vi "RT_Delta.vi"(4 "2812 -A Params In":T12={"Auto Range?"=FALSE, "Man / Selected\nRange"=enum."10mV", "Enable Digital\nFilter?"=FALSE, "Filter Type"=enum."Moving", "Filter Count"=10, "Filter\nWindow (%)"=0.01, "Enable Analog\nFilter?"=FALSE, "NPLCs"=5} {"Filter\nWindow (%)" min=0.0 max=10.0 step=0.01 format="%.2f"; "Filter Count" min=1 max=100; "NPLCs" min=1 max=10}, 6 "Delta Mode Params In":T1={"High Level (A)"=0.001, "Low Level (A)"=-0.001, "Delay (s)"=0.002, "Num Cycles Mode"=enum."Finite Count", "Finite Count"=10, "Abort On\nCompliance?"=FALSE, "Cold Swithing\nMode Enabled?"=FALSE} {"Finite Count" min=2 max=65536; "Low Level (A)" min=-0.105 max=0.0 format="%.3p"; "High Level (A)" min=0.0 max=0.105 format="%.3p"; "Delay (s)" min=0.001 max=9999.999 format="%.3f"}, 8 "error in (no error)":errorcluster, 11 "Resource In":refnum<visa-resource-name>) -> (0 "error out":errorcluster, 1 "Current (A)":sgl, 2 "Voltage (V)":dbl format="%0.2f", 3 "Resource Out (dupl)":refnum<visa-resource-name>)   [LabVIEW 2024]
uses:
  <instrlib>/Keithley 622x LV 2009/Configure/2182 -A/Low Level/Typedefs/KE2182 -- Voltage Ranges.ctl
  <instrlib>/Keithley 622x LV 2009/Configure/2182 -A/Low Level/Typedefs/KE2182 -- Filter Type.ctl
  <instrlib>/Keithley 622x LV 2009/Configure/2182 -A/Low Level/Typedefs/KE2182 -- Filter Count.ctl
  <instrlib>/Keithley 622x LV 2009/Configure/2182 -A/Low Level/Typedefs/KE2182 -- Filter Window.ctl
  <instrlib>/Keithley 622x LV 2009/Configure/2182 -A/Low Level/Typedefs/KE2182 -- NPLCs.ctl
  <instrlib>/Keithley 622x LV 2009/Configure/Delta PDelta DCon Modes/Typedefs/KE622x -- Delta Mode Params.ctl
  <instrlib>/Keithley 622x LV 2009/Configure/Delta PDelta DCon Modes/Low Level/Typedefs/KE622x -- Delta PDelta Mode High Level.ctl
  <instrlib>/Keithley 622x LV 2009/Configure/Delta PDelta DCon Modes/Low Level/Typedefs/KE622x -- Delta PDelta Mode Low Level.ctl
  <instrlib>/Keithley 622x LV 2009/Configure/Delta PDelta DCon Modes/Low Level/Typedefs/KE622x -- Delta DCon Mode Delay.ctl
  <instrlib>/Keithley 622x LV 2009/Configure/Delta PDelta DCon Modes/Low Level/Typedefs/KE622x -- Delta PDelta Mode Num Cycles Mode.ctl
  <instrlib>/Keithley 622x LV 2009/Configure/Delta PDelta DCon Modes/Low Level/Typedefs/KE622x -- Delta PDelta Mode Num Cycles.ctl
  <instrlib>/Keithley 622x LV 2009/Configure/Format/Typedefs/KE622x -- Optional Meas Elements.ctl
  <instrlib>/Keithley 622x LV 2009/Configure/Units/Typedefs/KE622x -- Voltage Meas Units.ctl
  <vilib>/Analysis/baseanly.llb/Mean (DBL).vi
  <instrlib>/Keithley 622x LV 2009/Keithley 622x.lvlib
  <vilib>/Analysis/NI_AALBase.lvlib
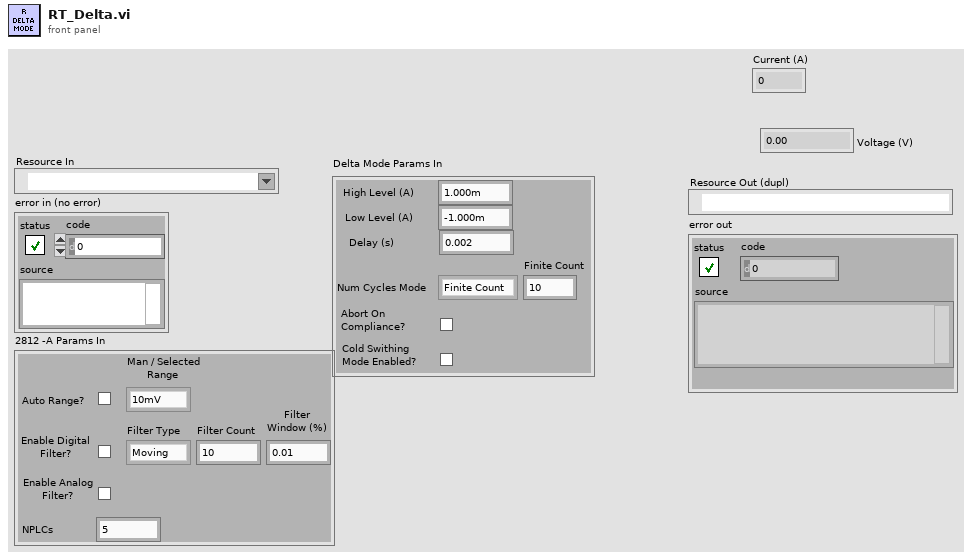
[diagram p1: front panel]
types:
  T1 = typedef "Keithley 622x.lvlib/KE622x -- Delta Mode Params.ctl" = cluster{"High Level (A)":T2, "Low Level (A)":T3, "Delay (s)":T4, "Num Cycles Mode":T5, "Finite Count":T6, "Abort On\nCompliance?":bool, "Cold Swithing\nMode Enabled?":bool}
  T2 = typedef "Keithley 622x.lvlib/KE622x -- Delta PDelta Mode High Level.ctl" = dbl
  T3 = typedef "Keithley 622x.lvlib/KE622x -- Delta PDelta Mode Low Level.ctl" = dbl
  T4 = typedef "Keithley 622x.lvlib/KE622x -- Delta DCon Mode Delay.ctl" = dbl
  T5 = typedef "Keithley 622x.lvlib/KE622x -- Delta PDelta Mode Num Cycles Mode.ctl" = enum16{"Finite Count", "Infinite"}
  T6 = typedef "Keithley 622x.lvlib/KE622x -- Delta PDelta Mode Num Cycles.ctl" = u32
  T7 = typedef "Keithley 622x.lvlib/KE2182 -- Voltage Ranges.ctl" = enum16{"10mV", "100mV", "1V", "10V", "100V"}
  T8 = typedef "Keithley 622x.lvlib/KE2182 -- Filter Type.ctl" = enum16{"Moving", "Repeat"}
  T9 = typedef "Keithley 622x.lvlib/KE2182 -- Filter Count.ctl" = u32
  T10 = typedef "Keithley 622x.lvlib/KE2182 -- Filter Window.ctl" = dbl
  T11 = typedef "Keithley 622x.lvlib/KE2182 -- NPLCs.ctl" = u32
  T12 = cluster{"Auto Range?":bool, "Man / Selected\nRange":T7, "Enable Digital\nFilter?":bool, "Filter Type":T8, "Filter Count":T9, "Filter\nWindow (%)":T10, "Enable Analog\nFilter?":bool, "NPLCs":T11}
  T13 = typedef "Keithley 622x.lvlib/KE622x -- Voltage Meas Units.ctl" = enum16{"Volts", "Ohms", "Watts", "Siemens"}
  T14 = typedef "Keithley 622x.lvlib/KE622x -- Optional Meas Elements.ctl" = cluster{"Timstamp?":bool, "Reading Num?":bool, "Source Value?":bool, "Compliance?":bool, "Average Voltage?":bool}
  T15 = typedef "Keithley 622x.lvlib/KE622x -- Trace Buf.ctl" = cluster{"Additional Valid Arrays":T14, "Reading Num":u32[], "Timestamp (secs)":sgl[], "Source Val (A)":sgl[], "Reading":sgl[], "Average Voltage (V)":sgl[], "Compliance?":bool[]}
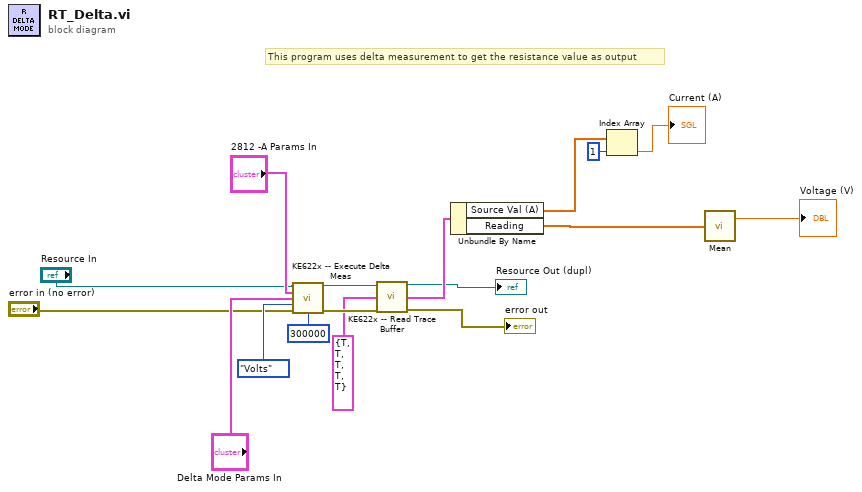
[diagram p0: block diagram]
diagram:
  # "This program uses delta measurement to get the resistance value as output"
  n1 = call <instrlib>:"KE622x -- Execute Delta Meas.vi"("Resource In"="Resource In", "2812 -A Params In"="2812 -A Params In", "Delta Mode Params In"="Delta Mode Params In", "Meas Units"=KE622x_--_Voltage_Meas_Units."Volts", "error in (no error)"="error in (no error)", "Timeout (20000 ms)"=u32 300000) -> ("Resource Out (dupl)"=w17:refnum<visa-resource-name>, "error out"=w16:errorcluster)  [unwired: 4 in, 4 out]
  n2 = call <instrlib>:"KE622x -- Read Trace Buffer.vi"("Resource In"=w17, "Meas Elements To Return"=T14 {"Timstamp?"=TRUE, "Reading Num?"=TRUE, "Source Value?"=TRUE, "Compliance?"=TRUE, "Average Voltage?"=TRUE}, "error in (no error)"=w16) -> ("Resource Out (dupl)"=→"Resource Out (dupl)":refnum<visa-resource-name>, "Trace Buf"=w14:T15, "error out"=→"error out":errorcluster)  [unwired: 10 in]
  n3 = Unbundle By Name(w14) -> ("Source Val (A)"=w5:sgl[], "Reading"=w1:sgl[])
  n4 = Index Array(array=w5, index=1) -> (element=→"Current (A)":sgl)
  n5 = call-poly <vilib>:"Mean.vi"("X"=w1) -> ("mean"=→"Voltage (V)":dbl)  [unwired: 1 out]
